vi "Definition.vi"(11 "NewEntityTemplate":refnum<class "NewEntityTemplate.lvclass">) -> (2 "Entity Definition":refnum<class "Type.lvclass">[](array[class]))   [LabVIEW 2020, in "NewEntityTemplate.lvclass"]
uses:
  NewEntityTemplate.lvclass
  NewEntityTemplate.lvclass/NewEntityTemplate.ctl
  Conditum/Columns/Type/Type.lvclass
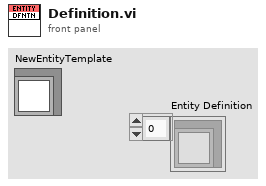
[diagram p1: front panel]
types:
  T1 = typedef "NewEntityTemplate.lvclass/Columns.ctl" = cluster{"Placeholder":refnum<class "Type.lvclass">}
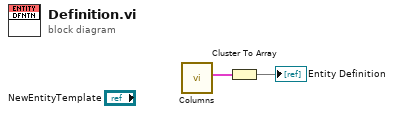
[diagram p0: block diagram]
diagram:
  n1 = call "Columns.vi"() -> ("Columns"=w2:T1)  [unwired: 11 in]
  n2 = Cluster To Array(cluster=w2) -> (array=→"Entity Definition":refnum<class "Type.lvclass">[])
